vi "Read_TPG300_sensor (SubVI).vi"(7 "Sensor CMD":string, 8 "error in (no error)":errorcluster, 11 "TCP Network Connection in":refnum<k5>) -> (0 "error out":errorcluster, 3 "connection ID out":refnum<k5>, 4 "out number":dbl, 5 "data out":string)   [LabVIEW 2015]
uses:
  <vilib>/Utility/error.llb/DialogType.ctl
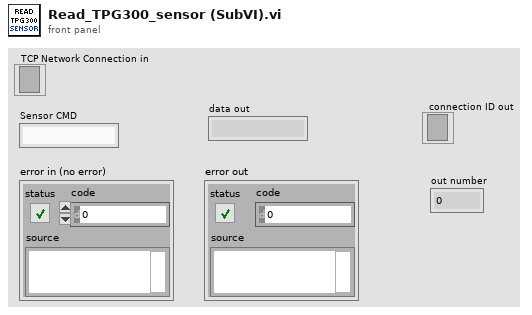
[diagram p1: front panel]
types:
  T1 = typedef "DialogType.ctl" = u16
  T2 = enum16{"Standard", "Buffered", "CRLF", "Immediate"}
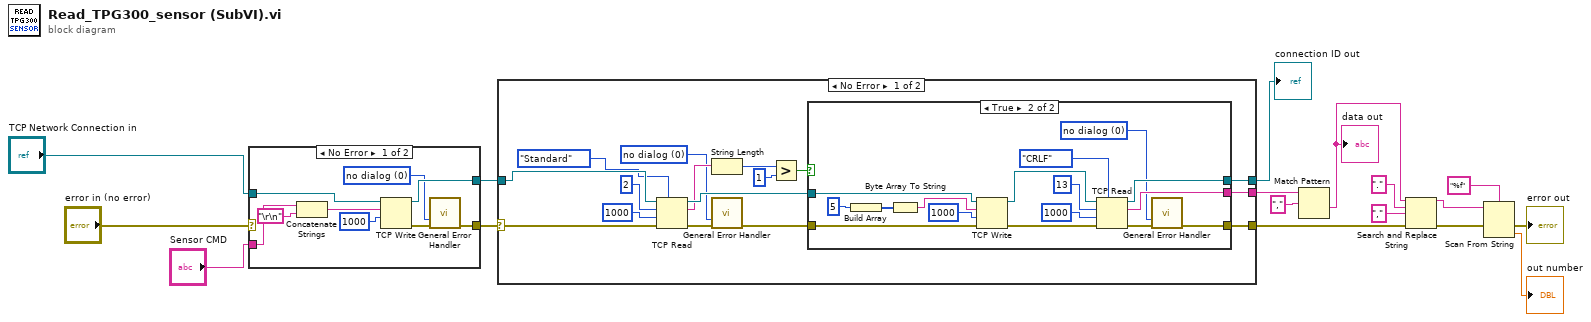
[diagram p0: block diagram]
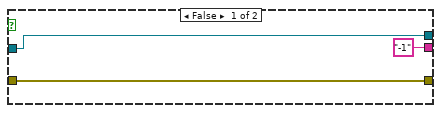
[diagram p2: hidden frame]
diagram:
  n1 = case shown="No Error" "error in (no error)" {
    selector: "error in (no error)" -> [_ w27]
    tunnel: [w20 w27] -> w4
    tunnel: [w26 w28] -> w17
    tunnel: "Sensor CMD" -> [w23 _]
    tunnel: "TCP Network Connection in" -> [w21 w28]
    frame No Error {
      w19 = T1 0 items=["no dialog", "OK message", "continue or stop message", "OK message + warnings", "continue/stop + warnings"] ("type of dialog (OK msg:1)")
      n2 = Concatenate Strings(w23, "\r\n") -> (w24:string)
      n3 = TCP Write(connection ID=w21, data in=w24, 9:1000 ("timeout ms (25000)")) -> (connection ID out=w26:refnum<k5>, error out=w18:errorcluster)  [unwired: 1 in, 1 out]
      n4 = call <vilib>:"General Error Handler.vi"("type of dialog (OK msg:1)"=w19, "error in (no error)"=w18) -> ("error out"=w20:errorcluster)  [unwired: 9 in, 4 out]
    }
    frame Error {
    }
  }
  n5 = case shown="No Error" w4 {
    selector: w4 -> [w32 w64]
    tunnel: w17 -> [w38 w65]
    tunnel: [w35 w65] -> w15
    tunnel: [w34 _] -> w9
    tunnel: [w33 w64] -> w8
    frame No Error {
      w30 = T1 0 items=["no dialog", "OK message", "continue or stop message", "OK message + warnings", "continue/stop + warnings"] ("type of dialog (OK msg:1)")
      n6 = TCP Read(connection ID=w38, bytes to read=2, error in (no error)=w32, 7:T2."Standard" ("mode (standard)"), 9:1000 ("timeout ms (25000)")) -> (connection ID out=w40:refnum<k5>, data out=w39:string, error out=w31:errorcluster)
      n7 = String Length(string=w39) -> (length=w42:i32)
      n8 = call <vilib>:"General Error Handler.vi"("type of dialog (OK msg:1)"=w30, "error in (no error)"=w31) -> ("error out"=w29:errorcluster)  [unwired: 9 in, 4 out]
      n9 = Greater?(x=w42, y=1) -> (0:w44:bool)
      n10 = case shown="True" w44 {
        tunnel: [w47 w49] -> w33
        tunnel: ["-1" ("data out") w55] -> w34
        tunnel: w29 -> [w47 w54]
        tunnel: w40 -> [w46 w53]
        tunnel: [w46 w51] -> w35
        frame False {
        }
        frame True {
          w48 = T1 0 items=["no dialog", "OK message", "continue or stop message", "OK message + warnings", "continue/stop + warnings"] ("type of dialog (OK msg:1)")
          n11 = Build Array(u8 5 ("millisecond multiple")) -> (w61:u8[])
          n12 = Byte Array To String(unsigned byte array=w61) -> (string=w60:string)
          n13 = TCP Write(connection ID=w53, data in=w60, error in (no error)=w54, 9:1000 ("timeout ms (25000)")) -> (connection ID out=w56:refnum<k5>, error out=w57:errorcluster)  [unwired: 1 out]
          n14 = TCP Read(connection ID=w56, bytes to read=13 ("timeout ms (25000)"), error in (no error)=w57, 7:T2."CRLF" ("mode (standard)"), 9:1000 ("timeout ms (25000)")) -> (connection ID out=w51:refnum<k5>, data out=w55:string, error out=w50:errorcluster)
          n15 = call <vilib>:"General Error Handler.vi"("type of dialog (OK msg:1)"=w48, "error in (no error)"=w50) -> ("error out"=w49:errorcluster)  [unwired: 9 in, 4 out]
        }
      }
    }
    frame Error {
    }
  }
  "connection ID out" <- w15
  n16 = Match Pattern(string=w9, regular expression=",") -> (after substring=w5:string)  [unwired: 1 in, 3 out]
  "data out" <- w5
  n17 = Search and Replace String(input string=w5, search string=".", replace string="," ("replace string (\"\")"), error in=w8) -> (result string=w14:string, error out=w7:errorcluster)  [unwired: 4 in, 2 out]
  n18 = Scan From String(format string="%f", input string=w14, error in=w7) -> (error out=→"error out":errorcluster, output 1=→"out number":dbl)  [unwired: 2 in, 2 out]
